vi "read_write.vi"() -> ()   [LabVIEW 2022 SP3]
uses:
  Library/dxl_x64_c.lvlib
panel:
  out "dynamixel_comm_result":string
  out "dynamixel_error":string
  in  "device_name":string="COM1"
  in  "ADDR_PRO_\nPRESENT_POSITION":u16=132
  in  "ADDR_PRO_\nGOAL_POSITION":u16=116
  in  "ADDR_PRO_\nTORQUE_ENABLE":u16=64
  out "protocol_version":dbl=2.0
  out "value : PRO (knob)\npresent position":i32(knob) scale=150000.0..-150000.0
  in  "terminate":bool
  out "port_num":i32
  in  "value : PRO (dial)\ngoal position":i32(knob) scale=150000.0..-150000.0
  in  "dynamixel_id":u8=1
  in  "baud_rate":i32=57600
  # "/*******************************************************************************\n* Copyright (c) 2016, ROBOTIS CO., LTD.\n* All rights reserved.\n*\n* Redistribution and use in source and binary forms, with or without\n* modification, are permitted provided that the following conditions are met:\n*\n* * Redistributions of source code must retain the above copyright notice, this\n*   list of conditions and the following disclaimer.\n*\n* * Redistributions in binary form must reproduce the above copyright notice,\n*   this list of conditions and the following disclaimer in the documentation\n*   and/or other materials provided with the distribution.\n*\n* * Neither the name of ROBOTIS nor the names of its\n*   contributors may be used to endorse or promote products derived from\n*   this software without specific prior written permission.\n*\n* THIS SOFTWARE IS PROVIDED BY THE COPYRIGHT HOLDERS AND CONTRIBUTORS \"AS IS\"\n* AND ANY EXPRESS OR IMPLIED WARRANTIES, INCLUDING, BUT NOT LIMITED TO, THE\n* IMPLIED WARRANTIES OF MERCHANTABILITY AND FITNESS FOR A PARTICULAR PURPOSE ARE\n* DISCLAIMED. IN NO EVENT SHALL THE COPYRIGHT HOLDER OR CONTRIBUTORS BE LIABLE\n* FOR ANY DIRECT, INDIRECT, INCIDENTAL, SPECIAL, EXEMPLARY, OR CONSEQUENTIAL\n* DAMAGES (INCLUDING, BUT NOT LIMITED TO, PROCUREMENT OF SUBSTITUTE GOODS OR\n* SERVICES; LOSS OF USE, DATA, OR PROFITS; OR BUSINESS INTERRUPTION) HOWEVER\n* CAUSED AND ON ANY THEORY OF LIABILITY, WHETHER IN CONTRACT, STRICT LIABILITY,\n* OR TORT (INCLUDING NEGLIGENCE OR OTHERWISE) ARISING IN ANY WAY OUT OF THE USE\n* OF THIS SOFTWARE, EVEN IF ADVISED OF THE POSSIBILITY OF SUCH DAMAGE.\n*******************************************************************************/\n\n/* Author: Ryu Woon Jung (Leon) */"
  # "Available Dynamixel model on this example : All models using Protocol 2.0\nThis example is designed for using a Dynamixel PRO 54-200, and an USB2DYNAMIXEL.\nTo use another Dynamixel model, such as X series, see their details in E-Manual(support.robotis.com) \n   and edit \"numeric control\"s seen left with \"Edit Text\" tool.\nBe sure that Dynamixel PRO properties are already set as %% ID : 1 / Baudnum : 1 (Baudrate : 57600)\n\n1. Run example by click above \"Run\" button (below \"Edit\" menu).\n2. Drag \"dial\" then you may see the Dynamixel and \"knob\" rotating\n3. To finish the example, press \"terminate\" button."
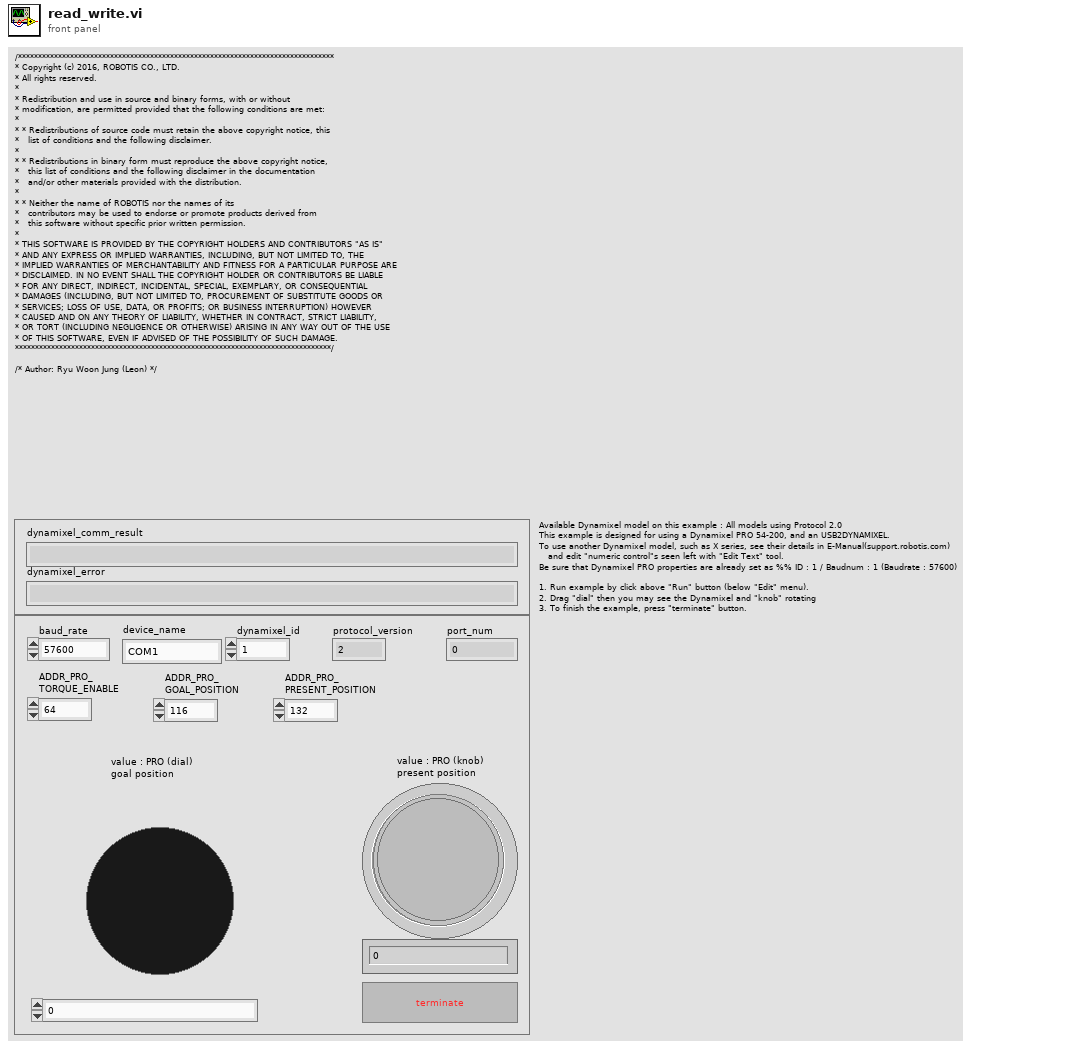
[diagram p1: front panel]
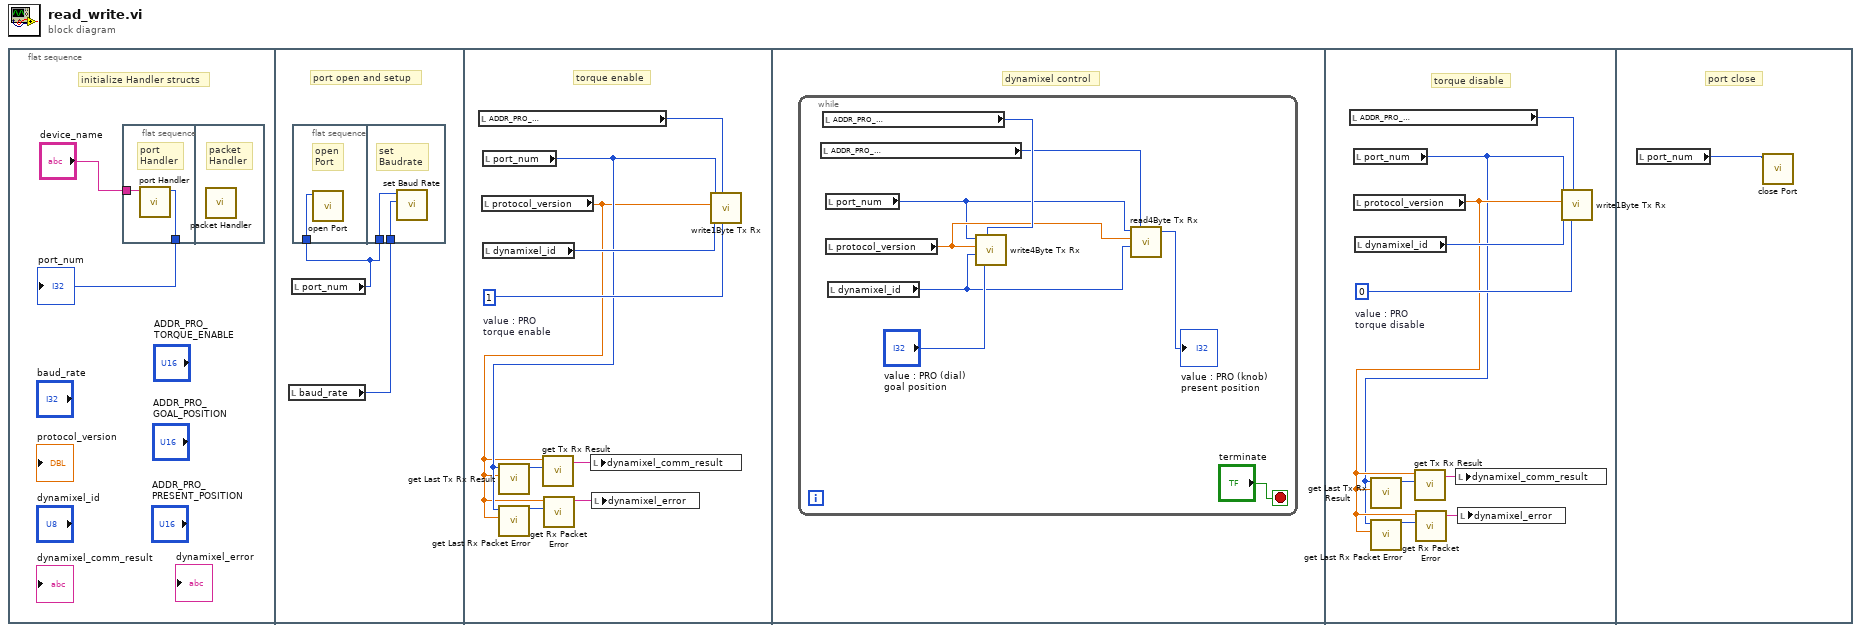
[diagram p0: block diagram]
diagram:
  n1 = flat-sequence {
    frame #0 {
      # "initialize Handler structs"
      n2 = flat-sequence {
        tunnel: [w4] -> w2
        tunnel: "device_name" -> [w3]
        frame #0 {
          # "port\nHandler"
          n3 = call "port Handler.vi"("port_name"=w3) -> ("function return"=w4:i32)  [unwired: 9 in, 1 out]
        }
        frame #1 {
          # "packet\nHandler"
          n4 = call "packet Handler.vi"() -> ()  [unwired: 11 in, 1 out]
        }
      }
      "port_num" <- w2
    }
    frame #1 {
      # "port open and setup"
      n5 = local read "baud_rate"() -> (w5:i32)
      n6 = local read "port_num"() -> (w6:i32)
      n7 = flat-sequence {
        tunnel: w6 -> [w7]
        tunnel: w6 -> [w9]
        tunnel: w5 -> [w8]
        frame #0 {
          # "open\nPort"
          n8 = call "open Port.vi"("port_num"=w7) -> ()  [unwired: 9 in, 2 out]
        }
        frame #1 {
          # "set\nBaudrate"
          n9 = call "set Baud Rate.vi"("baudrate"=w8, "port_num"=w9) -> ()  [unwired: 8 in, 2 out]
        }
      }
    }
    frame #2 {
      w18 = 1  # value : PRO torque enable
      # "torque enable"
      n10 = local read "ADDR_PRO_\nTORQUE_ENABLE"() -> (w16:u16)
      n11 = local read "protocol_version"() -> (w12:dbl)
      n12 = local read "port_num"() -> (w13:i32)
      n13 = local read "dynamixel_id"() -> (w17:u8)
      n14 = call "get Last Tx Rx Result.vi"("protocol_version"=w12, "port_num"=w13) -> ("function return"=w15:i32)  [unwired: 8 in, 1 out]
      n15 = call "get Last Rx Packet Error.vi"("protocol_version"=w12, "port_num"=w13) -> ("function return"=w14:u8)  [unwired: 8 in, 1 out]
      n16 = call "get Tx Rx Result.vi"("result"=w15, "protocol_version"=w12) -> ("function return"=w10:string)  [unwired: 8 in, 1 out]
      n17 = call "get Rx Packet Error.vi"("error"=w14, "protocol_version"=w12) -> ("function return"=w11:string)  [unwired: 8 in, 1 out]
      n18 = local write "dynamixel_comm_result"(w10) -> ()
      n19 = local write "dynamixel_error"(w11) -> ()
      n20 = call "write1Byte Tx Rx.vi"("data"=w18, "address"=w16, "id"=w17, "protocol_version"=w12, "port_num"=w13) -> ()  [unwired: 6 in, 1 out]
    }
    frame #3 {
      # "dynamixel control"
      n21 = while {
        stop <- "terminate" stop-if-true
        n22 = local read "ADDR_PRO_\nPRESENT_POSITION"() -> (w20:u16)
        n23 = local read "ADDR_PRO_\nGOAL_POSITION"() -> (w25:u16)
        n24 = local read "port_num"() -> (w21:i32)
        n25 = local read "protocol_version"() -> (w22:dbl)
        n26 = local read "dynamixel_id"() -> (w23:u8)
        n27 = call "write4Byte Tx Rx.vi"("data"="value : PRO (dial)\ngoal position", "address"=w25, "id"=w23, "protocol_version"=w22, "port_num"=w21) -> ()  [unwired: 6 in, 1 out]
        n28 = call "read4Byte Tx Rx.vi"("address"=w20, "id"=w23, "protocol_version"=w22, "port_num"=w21) -> ("function return"=→"value : PRO (knob)\npresent position":u32)  [unwired: 6 in, 1 out]
      }
    }
    frame #4 {
      w34 = 0  # value : PRO torque disable
      # "torque disable"
      n29 = local read "ADDR_PRO_\nTORQUE_ENABLE"() -> (w33:u16)
      n30 = local read "port_num"() -> (w29:i32)
      n31 = local read "protocol_version"() -> (w30:dbl)
      n32 = local read "dynamixel_id"() -> (w35:u8)
      n33 = call "get Last Tx Rx Result.vi"("protocol_version"=w30, "port_num"=w29) -> ("function return"=w31:i32)  [unwired: 8 in, 1 out]
      n34 = call "get Last Rx Packet Error.vi"("protocol_version"=w30, "port_num"=w29) -> ("function return"=w32:u8)  [unwired: 8 in, 1 out]
      n35 = call "get Tx Rx Result.vi"("result"=w31, "protocol_version"=w30) -> ("function return"=w28:string)  [unwired: 8 in, 1 out]
      n36 = call "get Rx Packet Error.vi"("error"=w32, "protocol_version"=w30) -> ("function return"=w27:string)  [unwired: 8 in, 1 out]
      n37 = local write "dynamixel_comm_result"(w28) -> ()
      n38 = local write "dynamixel_error"(w27) -> ()
      n39 = call "write1Byte Tx Rx.vi"("data"=w34, "address"=w33, "id"=w35, "protocol_version"=w30, "port_num"=w29) -> ()  [unwired: 6 in, 1 out]
    }
    frame #5 {
      # "port close"
      n40 = local read "port_num"() -> (w36:i32)
      n41 = call "close Port.vi"("port_num"=w36) -> ()  [unwired: 10 in, 1 out]
    }
  }
